vi "Count Logger States.vi"(8 "error in (no error)":errorcluster, 11 "Log Manager Module in":refnum<class "Log Manager Module.lvclass">) -> (0 "error out":errorcluster, 2 "Logger State Counts":map{T1, i32}(c390), 3 "Log Manager Module out":refnum<class "Log Manager Module.lvclass">)   [LabVIEW 2020, in "VolatusData.lvlib" / "Log Manager Module.lvclass"]
uses:
  Log Manager Module.lvclass
  Log Manager Module.lvclass/Log Manager Module.ctl
  <vilib>/Utility/miscctls.llb/LVMapReplaceAction.ctl
  Logger State.ctl
  VolatusData.lvlib
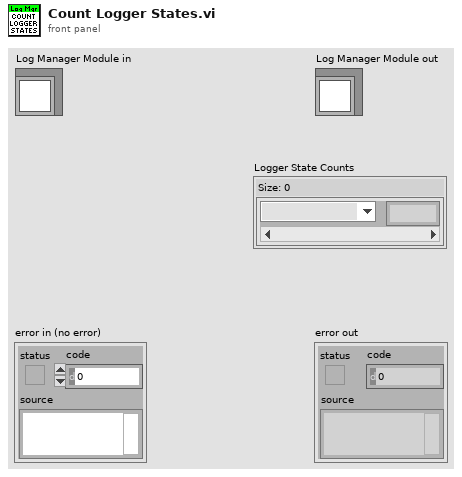
[diagram p1: front panel]
types:
  T1 = typedef "VolatusData.lvlib/Logger State.ctl" = enum16{"Unknown", "Idle", "Preparing", "Ready", "Logging", "Stopping"}
  T2 = typedef "VolatusData.lvlib/Log Manager Module.lvclass/Logger.ctl" = cluster{"ID":string, "MsgQ":refnum<class "MessageQ.lvclass">, "State":T1}
  T3 = typedef "LVMapReplaceAction.ctl" = enum32{"Modify Entry only if found", "Add or Modify Entry", "Delete Entry"}
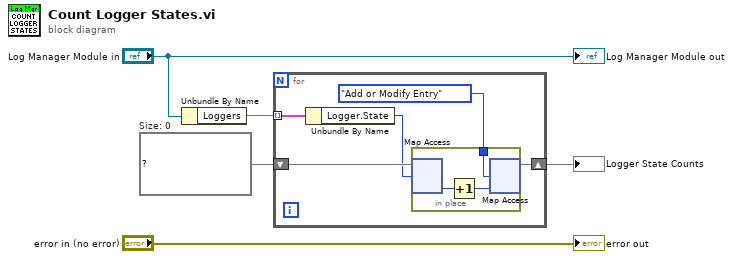
[diagram p0: block diagram]
diagram:
  w4 = map{T1, i32} {}  # Size: 0
  n1 = Unbundle By Name("Log Manager Module in") -> ("Loggers"=w3:map{string, T2})
  n2 = for {
    tunnel: w3 -> [w10] mode=indexing
    shift-right: [w6] -> w1
    shift-left: w4 -> [w9]
    n3 = Unbundle By Name(w10) -> ("Logger.State"=w8:T1)
    n4 = in-place {
      in-place-border: LVMapReplaceAction."Add or Modify Entry" ("action") -> [w11]
      n5 = in-place-map #1(w9, w8) -> (w13:i32)  [unwired: 1 in, 1 out]
      n6 = Increment(x=w13) -> (x+1=w12:i32)
      n7 = in-place-map #1(w12, w11) -> (w6:map{T1, i32})  [unwired: 2 out]
    }
  }
  "Logger State Counts" <- w1
  "error out" <- "error in (no error)"
  "Log Manager Module out" <- "Log Manager Module in"
